vi "TP program2.vi"() -> (1 "布尔 2":bool, 2 "order":string caption="FileName:")   [LabVIEW 2018]
panel:
  in  "Bar":bool
  out "error out":errorcluster caption="错误输出"
  in  "error in (no error)":errorcluster caption="错误输入（无错误）"
  out "布尔":bool
  out "Row":i32
  in  "Cancel":bool
  in  "OK":bool
  in  "Program list":i32(listbox)
  # "TestProgramSelet"
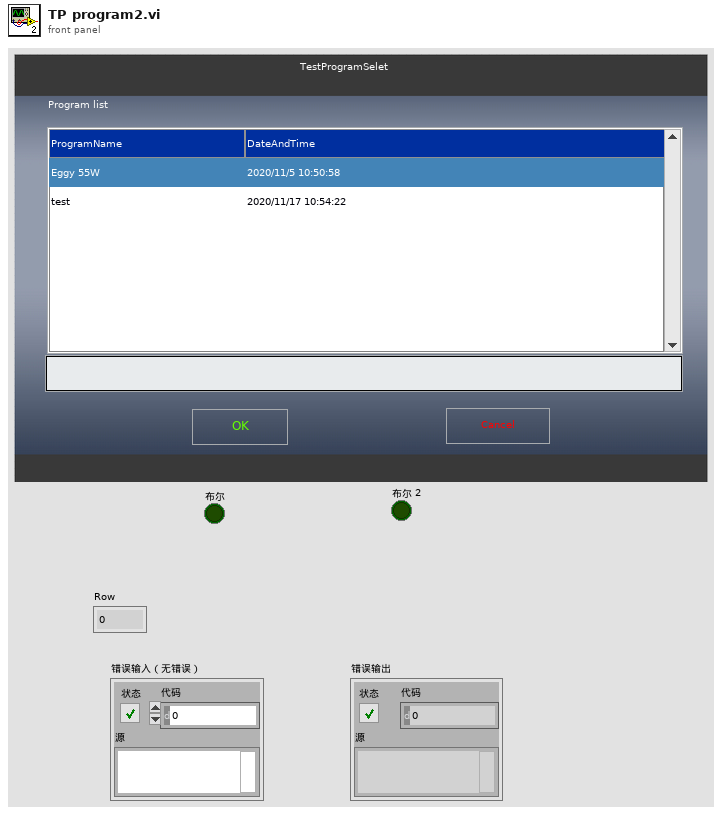
[diagram p1: front panel]
types:
  T1 = typedef "Window Refnum.ctl" = refnum<k1>
  T2 = typedef "LVPoint32TypeDef.ctl" = cluster{"Horizontal":i32, "Vertical":i32}
  T3 = typedef "LVRowAndColumnTypeDef.ctl" = cluster{"Row":i32, "Column":i32}
  T4 = typedef "Window Rectangle.ctl" = cluster{"left":i16, "top":i16, "right":i16, "bottom":i16}
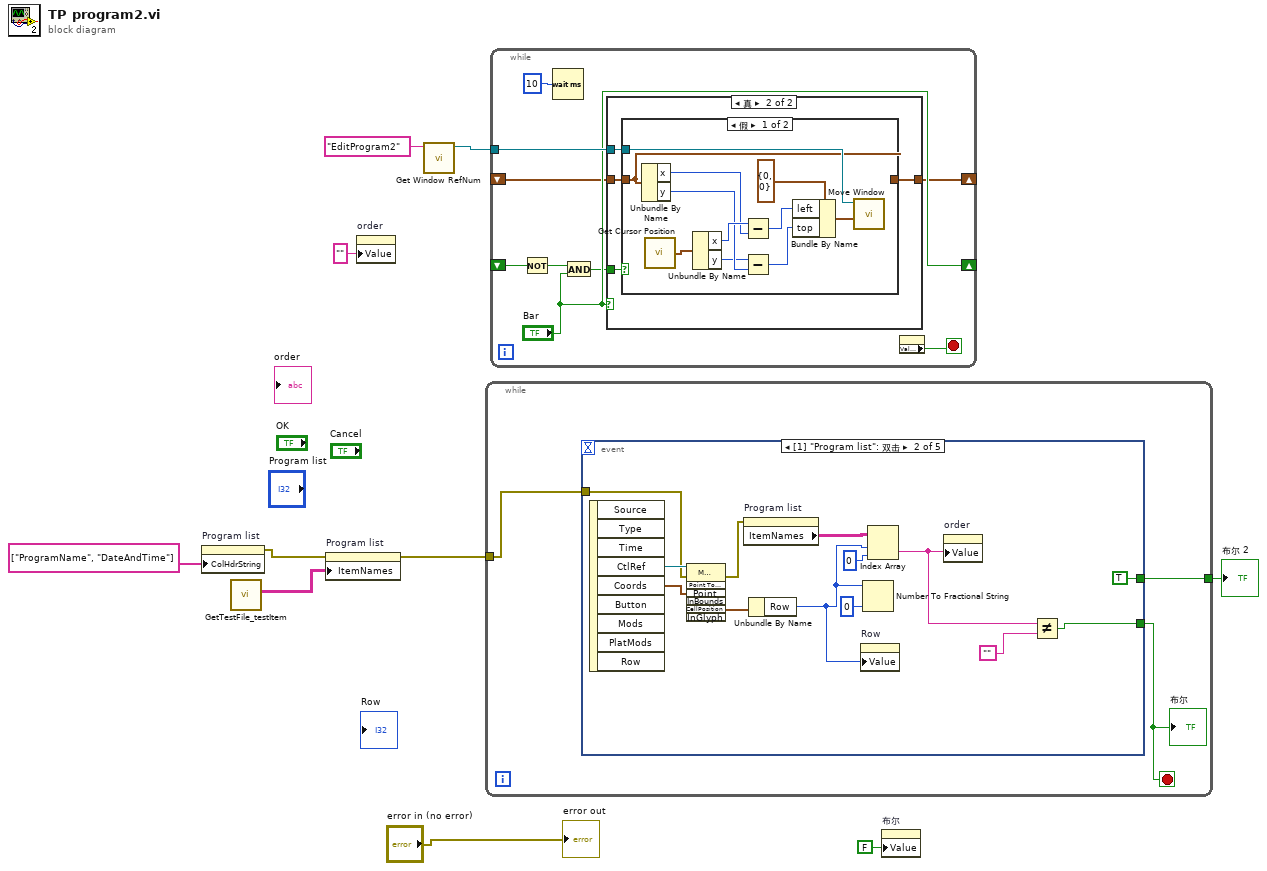
[diagram p0: block diagram]
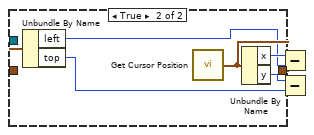
[diagram p3: hidden frame]
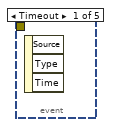
[diagram p4: hidden frame]
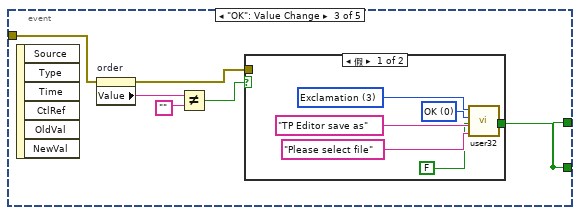
[diagram p5: hidden frame]
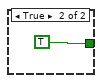
[diagram p6: hidden frame]
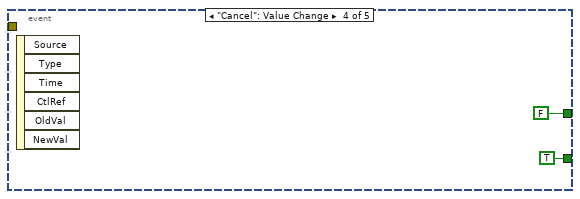
[diagram p7: hidden frame]
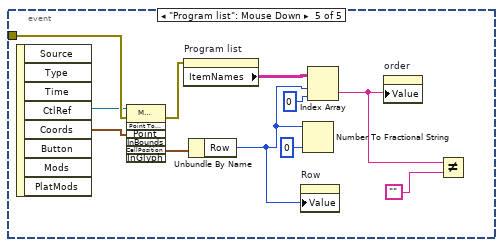
[diagram p8: hidden frame]
diagram:
  n1 = property on="Program list" class="MCListbox (严格)"("ColHdrString"=string[] ["ProgramName", "DateAndTime"] ("Column Header Strings[]")) -> (error out=w8:errorcluster)  [unwired: 2 in, 1 out]
  n2 = call "GetTestFile_testItem.vi"() -> ("转置的数组"=w10:string[][])  [unwired: 10 in, 1 out]
  n3 = property on="Program list" class="MCListbox (严格)"(error in=w8, "ItemNames"=w10) -> (error out=w7:errorcluster)  [unwired: 1 in, 1 out]
  n4 = property on="order" class="Str"("Value"="" ("order")) -> ()  [unwired: 2 in, 2 out]
  n5 = call "Get Window RefNum.vi"("window name (\"\")"="EditProgram2" ("window name (\"\")")) -> ("window refnum (NaWR)"=w6:T1)  [unwired: 1 in, 7 out]
  n6 = while {
    tunnel: w7 -> [w13]
    tunnel: [w11] -> w1
    stop <- w12 stop-if-true
    n7 = event shown="[1] \"Program list\": 双击" {
      selector: _ -> [_ _ _ _ _]
      dyn-events: _ -> [_ _ _ _ _]
      timeout: _ -> [_ _ _ _ _]
      tunnel: w13 -> [_ w18 w32 _ w45]
      tunnel: [_ w16 w27 TRUE _] -> w12
      tunnel: [_ TRUE w27 FALSE _] -> w11
      event Timeout {
        n8 = event-data() -> ()  [unwired: 1 in, 3 out]
      }
      event "Program list": Double Click {
        n9 = event-data() -> ("CtlRef"=w26:refnum<vi>, "Coords"=w25:T2)  [unwired: 1 in, 7 out]
        n10 = invoke class="MCListbox (严格)" method="Point To Row Column"(reference=w26, error in=w18, "Point"=w25) -> (error out=w19:errorcluster, "CellPosition"=w22:T3)  [unwired: 4 in, 5 out]
        n11 = property on="Program list" class="MCListbox (严格)"(error in=w19) -> ("ItemNames"=w21:string[][])  [unwired: 1 in, 2 out]
        n12 = Unbundle By Name(w22) -> ("Row"=w20:i32)
        n13 = property on="Row" class="DigNum (严格)"("Value"=w20) -> ()  [unwired: 2 in, 2 out]
        n14 = Number To Fractional String(number=w20, precision (6)=i16 0 ("精度(6)")) -> ()  [unwired: 2 in, 1 out]
        n15 = Index Array(array=w21, index (row)=w20, index (col)=0 ("disabled index (col)")) -> (element=w15:string)
        n16 = property on="order" class="Str"("Value"=w15) -> ()  [unwired: 2 in, 2 out]
        n17 = Not Equal?(x=w15, y="") -> (x != y?=w16:bool)
      }
      event "OK": Value Change {
        n18 = event-data() -> ()  [unwired: 1 in, 6 out]
        n19 = property on="order" class="Str"(error in=w32) -> (error out=w29:errorcluster, "Value"=w30:string)  [unwired: 1 in, 1 out]
        n20 = Not Equal?(x=w30, y="") -> (x != y?=w28:bool)
        n21 = case shown="假" w28 {
          tunnel: [FALSE TRUE] -> w27
          tunnel: w29 -> [_ _]
          frame False {
            w36 = u16 0 items=["OK", "OK+Cancel", "Abort+Retry+Ignore", "Yes+ON+Cancel", "Yes+No", "Retry+Cancel", "Cancel+Retry+Continue"] ("Buttons")
            w37 = u16 3 items=["None", "Critical", "Question", "Exclamation", "Infomation"] ("Icon")
            n22 = call "user32.vi"("Icon"=w37, "Buttons"=w36, "Ipcaption"="TP Editor save as", "IP Text"="Please select file") -> ()  [unwired: 2 out]
          }
          frame True {
          }
        }
      }
      event "Cancel": Value Change {
        n23 = event-data() -> ()  [unwired: 1 in, 6 out]
      }
      event "Program list": Mouse Down {
        n24 = event-data() -> ("CtlRef"=w44:refnum<vi>, "Coords"=w43:T2)  [unwired: 1 in, 6 out]
        n25 = invoke class="MCListbox (严格)" method="Point To Row Column"(reference=w44, error in=w45, "Point"=w43) -> (error out=w48:errorcluster, "CellPosition"=w51:T3)  [unwired: 4 in, 5 out]
        n26 = property on="Program list" class="MCListbox (严格)"(error in=w48) -> ("ItemNames"=w50:string[][])  [unwired: 1 in, 2 out]
        n27 = Unbundle By Name(w51) -> ("Row"=w49:i32)
        n28 = property on="Row" class="DigNum (严格)"("Value"=w49) -> ()  [unwired: 2 in, 2 out]
        n29 = Number To Fractional String(number=w49, precision (6)=i16 0 ("精度(6)")) -> ()  [unwired: 2 in, 1 out]
        n30 = Index Array(array=w50, index (row)=w49, index (col)=0 ("disabled index (col)")) -> (element=w42:string)
        n31 = property on="order" class="Str"("Value"=w42) -> ()  [unwired: 2 in, 2 out]
        n32 = Not Equal?(x=w42, y="") -> ()  [unwired: 1 out]
      }
    }
    "布尔" <- w12
  }
  "布尔 2" <- w1
  n33 = while {
    shift-left: _ -> [w54]
    shift-right: [w55] -> _
    shift-left: _ -> [w58]
    shift-right: ["Bar"] -> _
    tunnel: w6 -> [w59]
    stop <- w52 stop-if-true
    n34 = Not(x=w58) -> (.not. x?=w57:bool)
    n35 = Wait (ms)(milliseconds to wait=u32 10) -> ()  [unwired: 1 out]
    n36 = And(x=w57, y="Bar") -> (x .and. y?=w53:bool)
    n37 = case shown="真" "Bar" {
      tunnel: w59 -> [_ w65]
      tunnel: [w61 w64] -> w55
      tunnel: w54 -> [w61 w62]
      tunnel: w53 -> [_ w63]
      frame False {
      }
      frame True {
        n38 = case shown="假" w63 {
          tunnel: w65 -> [w71 w87]
          tunnel: [w66 w77] -> w64
          tunnel: w62 -> [w66 _]
          frame False {
            n39 = Unbundle By Name(w66) -> ("x"=w74:i16, "y"=w73:i16)
            n40 = call "Get Cursor Position.vi"() -> ("cursor position"=w76:cluster{"x":i16, "y":i16})
            n41 = Unbundle By Name(w76) -> ("x"=w75:i16, "y"=w72:i16)
            n42 = Subtract(x=w75, y=w74) -> (x-y=w68:i16)
            n43 = Subtract(x=w72, y=w73) -> (x-y=w69:i16)
            n44 = Bundle By Name(cluster=cluster{"left":i16, "top":i16} {"left"=0, "top"=0} ("new position (0,0)"), "left"=w68, "top"=w69) -> (w67:cluster{"left":i16, "top":i16})
            n45 = call "Move Window.vi"("new position (0,0)"=w67, "window refnum (NaWR)"=w71) -> ()  [unwired: 2 in, 4 out]
          }
          frame True {
            n46 = call "Get Window Rectangle.vi"("window refnum (NaWR)"=w87) -> ("window rect"=w86:T4)  [unwired: 1 in, 5 out]
            n47 = call "Extract Window Origin.vi"("window rect"=w86) -> ("window origin"=w85:cluster{"left":i16, "top":i16})  [unwired: 1 out]
            n48 = Unbundle By Name(w85) -> ("left"=w82:i16, "top"=w81:i16)
            n49 = call "Get Cursor Position.vi"() -> ("cursor position"=w84:cluster{"x":i16, "y":i16})
            n50 = Unbundle By Name(w84) -> ("x"=w83:i16, "y"=w80:i16)
            n51 = Subtract(x=w83, y=w82) -> (x-y=w78:i16)
            n52 = Subtract(x=w80, y=w81) -> (x-y=w79:i16)
            n53 = Bundle By Name(cluster=w84, "x"=w78, "y"=w79) -> (w77:cluster{"x":i16, "y":i16})
          }
        }
      }
    }
    n54 = property on="布尔" class="Bool (严格)"() -> ("Value"=w52:bool)  [unwired: 2 in, 2 out]
  }
  n55 = property on="布尔" class="Bool (严格)"("Value"=FALSE ("布尔")) -> ()  [unwired: 2 in, 2 out]
  "error out" <- "error in (no error)"
